vi "us_to_s.vi"(1 "Time / us":dbl) -> (0 "Time / s":dbl)   [LabVIEW 2023]
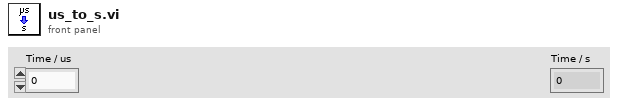
[diagram p1: front panel]
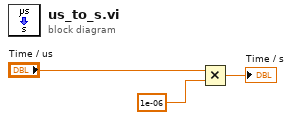
[diagram p0: block diagram]
diagram:
  n1 = Multiply(x="Time / us", y=1e-06) -> (x*y=→"Time / s":dbl)
